vi "1.Intro_GJE.vi"() -> ()   [LabVIEW 2018]
panel:
  out "X/Y":dbl
  in  "Y":i8
  out "Slide 3":dbl(slide) scale=0.0..9.0
  out "Slide 2":dbl(slide) scale=0.0..9.0
  out "Gauge":i8(knob) scale=0.0..9.0
  in  "X":i8
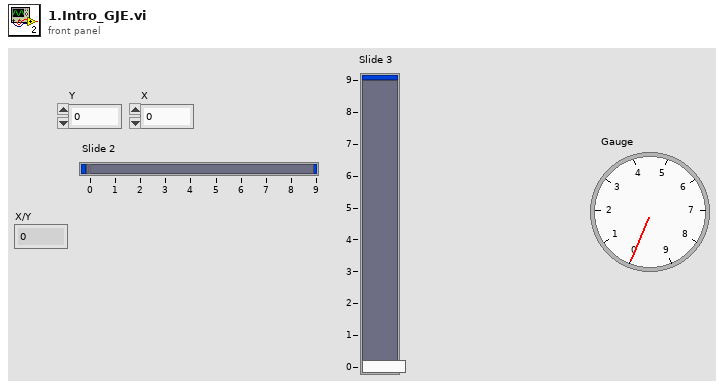
[diagram p1: front panel]
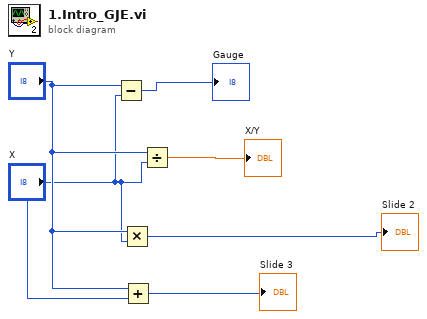
[diagram p0: block diagram]
diagram:
  n1 = Subtract(x="Y", y="X") -> (x-y=→"Gauge":i8)
  n2 = Multiply(x="Y", y="X") -> (x*y=→"Slide 2":i8)
  n3 = Add(x="Y", y="X") -> (x+y=→"Slide 3":i8)
  n4 = Divide(x="Y", y="X") -> (x/y=→"X/Y":dbl)
